vi "WPI_DriverStationLaptopDataCache.vi"(7 "LaptopCacheOp":T1, 11 "Laptop Data":u8[](array[numeric])) -> (3 "Laptop Data Out":u8[](array[numeric]))   [LabVIEW 2017]
doc: "This software is licensed. Open the labview\\readme\\WPI Robotics Library Open Source License.txt file for more information."
uses:
  <vilib>/Rock Robotics/WPI/DriverStation/WPI_DriverStationLaptopDataCacheOp.ctl
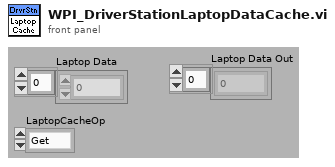
[diagram p1: front panel]
types:
  T1 = typedef "WPI_DriverStationLaptopDataCacheOp.ctl" = enum16{"Get", "Set", "Init"}
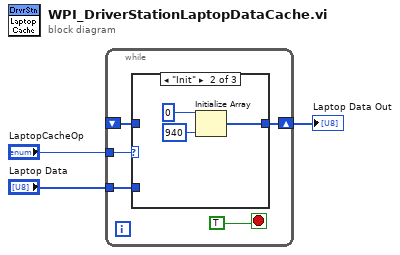
[diagram p0: block diagram]
diagram:
  n1 = while {
    shift-right: [w7] -> w1
    shift-left: _ -> [w6]
    tunnel: "LaptopCacheOp" -> [w8]
    tunnel: "Laptop Data" -> [w5]
    stop <- TRUE stop-if-true
    n2 = case shown="\"Init\"" w8 {
      tunnel: [w9 w10 w13] -> w7
      tunnel: w6 -> [_ _ w13]
      tunnel: w5 -> [w9 _ _]
      frame "Set", Default {
      }
      frame "Init" {
        n3 = Initialize Array(u8 0 ("element"), 940 ("dimension size")) -> (w10:u8[])
      }
      frame "Get" {
      }
    }
  }
  "Laptop Data Out" <- w1
